vi "subvi_randomarray.vi"(7 "original image":picture[][](array[picture]), 10 "Width/Height":i32, 11 "Element number":i32) -> (3 "random array":picture[][](array[picture]))   [LabVIEW 2014]
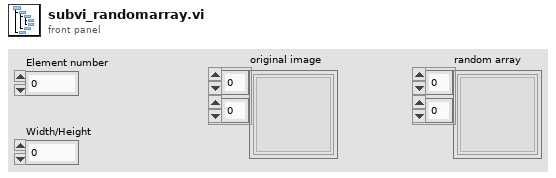
[diagram p1: front panel]
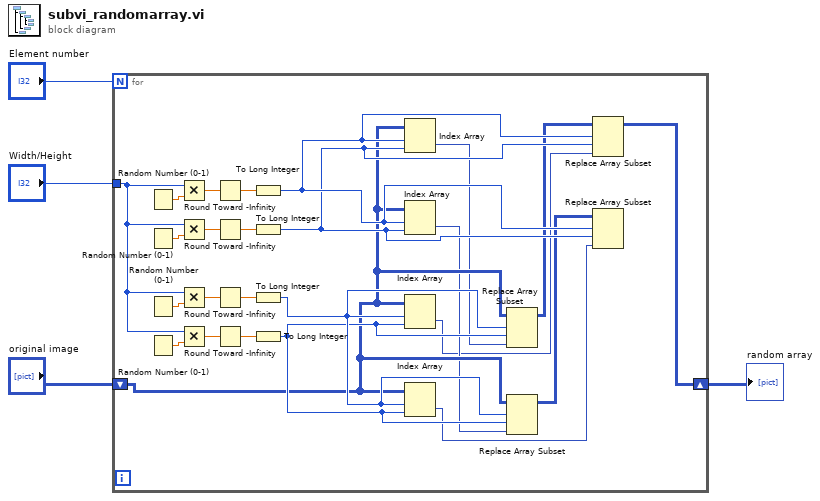
[diagram p0: block diagram]
diagram:
  n1 = for "Shuffle Array Elements" {
    N: "Element number" -> [_]
    tunnel: "Width/Height" -> [w21]
    shift-right: [w5] -> w2
    shift-left: "original image" -> [w12]
    n2 = Random Number (0-1)() -> (number: 0 to 1=w29:dbl)
    n3 = Random Number (0-1)() -> (number: 0 to 1=w26:dbl)
    n4 = Random Number (0-1)() -> (number: 0 to 1=w22:dbl)
    n5 = Random Number (0-1)() -> (number: 0 to 1=w25:dbl)
    n6 = Multiply(x=w21, y=w29) -> (x*y=w28:dbl)
    n7 = Multiply(x=w21, y=w26) -> (x*y=w27:dbl)
    n8 = Multiply(x=w21, y=w22) -> (x*y=w23:dbl)
    n9 = Multiply(x=w21, y=w25) -> (x*y=w24:dbl)
    n10 = Round Toward -Infinity(1:w28) -> (0:w17:dbl)
    n11 = Round Toward -Infinity(1:w27) -> (0:w18:dbl)
    n12 = Round Toward -Infinity(1:w23) -> (0:w19:dbl)
    n13 = Round Toward -Infinity(1:w24) -> (0:w20:dbl)
    n14 = To Long Integer(number=w17) -> (32bit integer=w16:i32)
    n15 = To Long Integer(number=w18) -> (32bit integer=w15:i32)
    n16 = To Long Integer(number=w19) -> (32bit integer=w14:i32)
    n17 = To Long Integer(number=w20) -> (32bit integer=w13:i32)
    n18 = Index Array(array=w12, index (row)=w16, index (col)=w15) -> (element=w11:picture)
    n19 = Index Array(array=w12, index (row)=w16, index (col)=w15) -> (element=w10:picture)
    n20 = Index Array(array=w12, index (row)=w14, index (col)=w13) -> (element=w8:picture)
    n21 = Index Array(array=w12, index (row)=w14, index (col)=w13) -> (element=w9:picture)
    n22 = Replace Array Subset(array=w12, new element=w11, index (row)=w14, index (col)=w13) -> (w7:picture[][])
    n23 = Replace Array Subset(array=w12, new element=w10, index (row)=w14, index (col)=w13) -> (w6:picture[][])
    n24 = Replace Array Subset(array=w7, new element=w8, index (row)=w16, index (col)=w15) -> (w5:picture[][])
    n25 = Replace Array Subset(array=w6, new element=w9, index (row)=w16, index (col)=w15) -> ()  [unwired: 1 out]
  }
  "random array" <- w2
